vi "Library Remote Call Error Merger.vi"(0 "call by reference node error":errorcluster, 11 "called VI error (no error)":errorcluster) -> (15 "error out":errorcluster)   [LabVIEW 2012]
doc: "This VI is designed for proper wiring and reporting of errors as generated by a remote \"Call by Reference\". When the call by reference node itself fails this indicates network or connection trouble and this VI will add some explanation to the error for the benefit of the user. If the call succeeded, but the called VI failed, the source is examined to see if the call was made to a different runtime (via a proxy VI). If so, the remote call chain is extended with the local call chain."
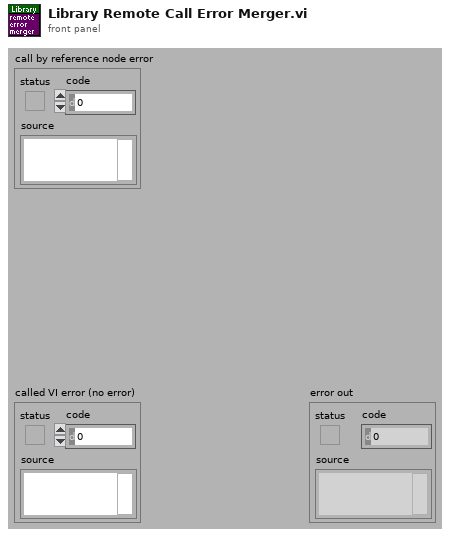
[diagram p1: front panel]
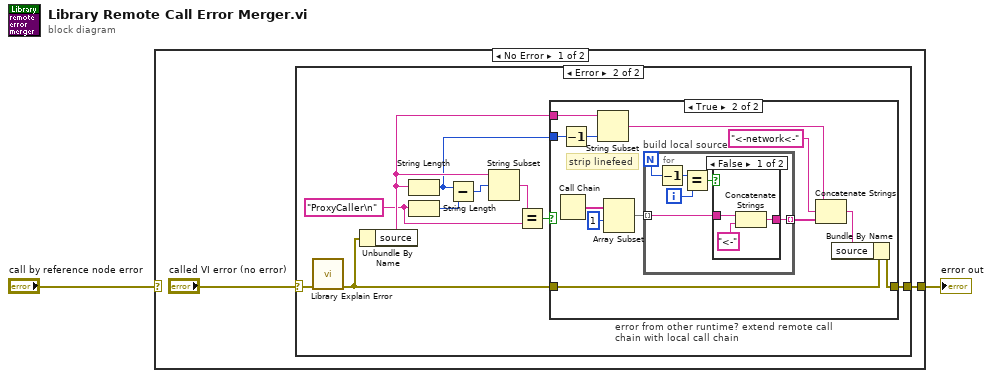
[diagram p0: block diagram]
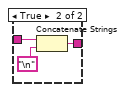
[diagram p4: hidden frame]
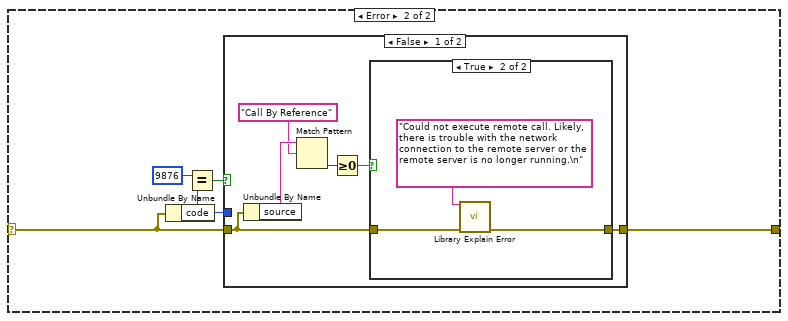
[diagram p5: hidden frame]
diagram:
  n1 = case shown="No Error" "call by reference node error" {
    selector: "call by reference node error" -> [_ w42]
    tunnel: [w3 w45] -> w2
    frame No Error {
      n2 = case shown="Error" "called VI error (no error)" {
        selector: "called VI error (no error)" -> [w5 w11]
        tunnel: [w5 w12] -> w3
        frame No Error {
        }
        frame Error {
          w7 = "ProxyCaller\n" ("x")
          n3 = call "Library Explain Error.vi"("error in (no error)"=w11) -> ("explained error"=w10:errorcluster)  [unwired: 14 in]
          n4 = Unbundle By Name(w10) -> ("source"=w13:string)
          n5 = String Length(string=w13) -> (length=w6:i32)
          n6 = String Length(string=w7) -> (length=w9:i32)
          n7 = Subtract(x=w6, y=w9) -> (x-y=w15:i32)
          n8 = String Subset(string=w13, offset (0)=w15) -> (substring=w8:string)  [unwired: 1 in]
          n9 = Equal?(x=w8, y=w7) -> (x = y?=w14:bool)
          n10 = case "error from other runtime? extend remote call chain with local call chain" shown="True" w14 {
            tunnel: w13 -> [_ w24]
            tunnel: w10 -> [w16 w22]
            tunnel: [w16 w21] -> w12
            tunnel: w6 -> [_ w20]
            frame False {
            }
            frame True {
              # "strip linefeed"
              n11 = Call Chain() -> (call chain=w28:string[])
              n12 = Decrement(x=w20) -> (x-1=w19:i32)
              n13 = String Subset(string=w24, length (rest)=w19) -> (substring=w18:string)  [unwired: 1 in]
              n14 = Array Subset(array=w28, index=1) -> (w27:string[])  [unwired: 1 in]
              n15 = for "build local source" {
                N -> [w34]
                tunnel: w27 -> [w30] mode=indexing
                tunnel: [w29] -> w25 mode=indexing
                i -> [w32]
                n16 = Decrement(x=w34) -> (x-1=w33:i32)
                n17 = Equal?(x=w33, y=w32) -> (x = y?=w31:bool)
                n18 = case shown="False" w31 {
                  tunnel: w30 -> [w36 w40]
                  tunnel: [w35 w38] -> w29
                  frame False {
                    n19 = Concatenate Strings(w36, "<-") -> (w35:string)
                  }
                  frame True {
                    n20 = Concatenate Strings(w40, "\n") -> (w38:string)
                  }
                }
              }
              n21 = Concatenate Strings(w18, "<-network<-", w25) -> (w23:string)
              n22 = Bundle By Name(cluster=w22, "source"=w23) -> (w21:errorcluster)
            }
          }
        }
      }
    }
    frame Error {
      n23 = Unbundle By Name(w42) -> ("code"=w44:i32)
      n24 = Equal?(x=9876, y=w44) -> (x = y?=w43:bool)
      n25 = case shown="False" w43 {
        tunnel: [w51 w56] -> w45
        tunnel: w44 -> [_ _]
        tunnel: w42 -> [w50 w56]
        frame False {
          n26 = Unbundle By Name(w50) -> ("source"=w49:string)
          n27 = Match Pattern(string=w49, regular expression="Call By Reference" ("search string")) -> (offset past match=w46:i32)  [unwired: 1 in, 3 out]
          n28 = Greater Or Equal To 0?(x=w46) -> (x >= 0?=w47:bool)
          n29 = case shown="True" w47 {
            tunnel: [w52 w55] -> w51
            tunnel: w50 -> [w52 w54]
            frame False {
            }
            frame True {
              n30 = call "Library Explain Error.vi"("explanation prefix (none)"="Could not execute remote call. Likely, there is trouble with the network connection to the remote server or the remote server is no longer running.\n" ("format string"), "error in (no error)"=w54) -> ("explained error"=w55:errorcluster)  [unwired: 13 in]
            }
          }
        }
        frame True {
          # "Already an explained error"
        }
      }
    }
  }
  "error out" <- w2
